vi "Test Clone Registration API.vi"() -> ()   [LabVIEW 2022 SP3, in "Serial-Com-Module.lvlib"]
doc: "Tester for the cloneable module registry VIs.\n_____\nBased on DQMH Project Template 6.1.0.94."
uses:
  Serial-Com-Module.lvlib
  Clone Registration.lvlib
panel:
  out "Empty?":bool
  out "First?":bool
  out "Module IDs":cluster{"Boolean":bool, "Numeric":i32}[](array[cluster])
  out "found?":bool
  out "replaced?":bool
  in  "Remove Module":bool
  in  "Add Module":bool
  in  "Module ID":i32
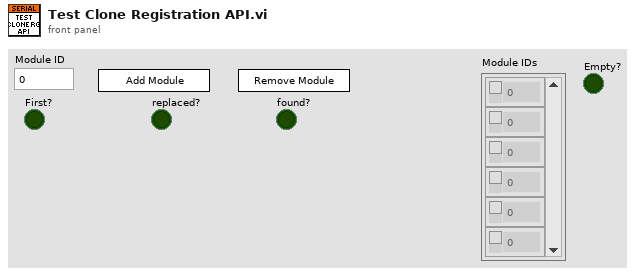
[diagram p1: front panel]
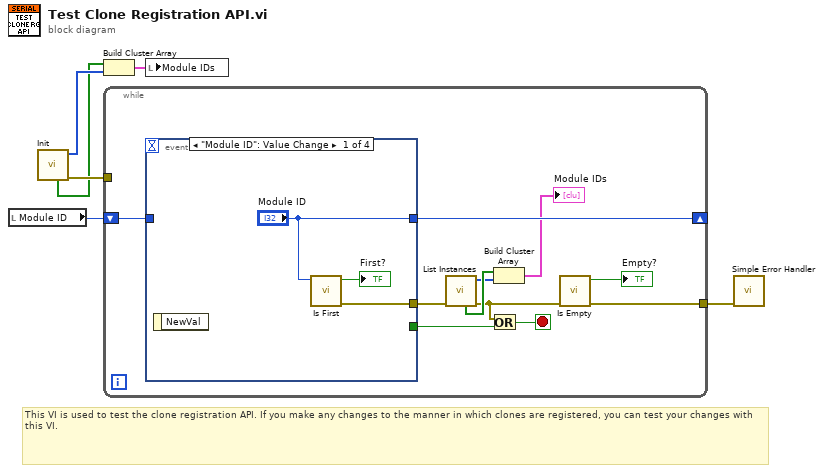
[diagram p0: block diagram]
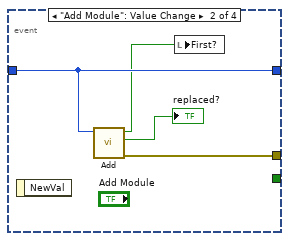
[diagram p2: hidden frame]
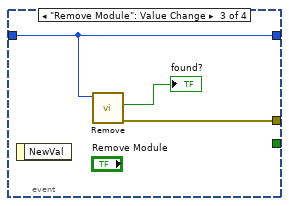
[diagram p3: hidden frame]
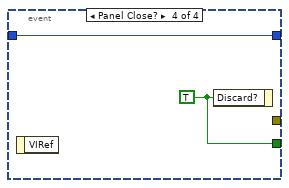
[diagram p4: hidden frame]
diagram:
  # "This VI is used to test the clone registration API. If you make any changes to the manner in which clones are registered, you can test your changes with this VI."
  n1 = local read "Module ID"() -> (w6:i32)
  n2 = call "Init.vi"() -> ("error out"=w2:errorcluster, "Module IDs"=w3:i32[], "First? (all)"=w1:bool[])  [unwired: 8 in, 1 out]
  n3 = Build Cluster Array(w1, w3) -> (w5:cluster{"First?":bool, "Module ID":i32}[])
  n4 = while {
    shift-right: [w16] -> _
    shift-left: w6 -> [w15]
    tunnel: w2 -> [_]
    tunnel: [w8] -> w4
    stop <- w14 stop-if-true
    n5 = event shown="[0] \"Module ID\": Value Change" {
      selector: _ -> [_ _ _ _]
      dyn-events: _ -> [_ _ _ _]
      timeout: _ -> [_ _ _ _]
      tunnel: [_ _ _ w29] -> w17
      tunnel: ["Module ID" w24 w25 w28] -> w16
      tunnel: w15 -> [_ w24 w25 w28]
      tunnel: [w18 w21 w27 _] -> w10
      event "Module ID": Value Change {
        n6 = event-data() -> ()  [unwired: 1 in, 1 out]
        n7 = call "Is First.vi"("Module ID"="Module ID") -> ("error out"=w18:errorcluster, "First?"=→"First?":bool)  [unwired: 9 in]
      }
      event "Add Module": Value Change {
        n8 = event-data() -> ()  [unwired: 1 in, 1 out]
        n9 = call "Add.vi"("Module ID"=w24) -> ("error out"=w21:errorcluster, "replaced?"=→"replaced?":bool, "First?"=w23:bool)  [unwired: 8 in]
        n10 = local write "First?"(w23) -> ()
      }
      event "Remove Module": Value Change {
        n11 = event-data() -> ()  [unwired: 1 in, 1 out]
        n12 = call "Remove.vi"("Module ID"=w25) -> ("error out"=w27:errorcluster, "empty"=→"found?":bool)  [unwired: 9 in]
      }
      event Panel Close? {
        w29 = TRUE ("Discard?")
        n13 = event-data() -> ()  [unwired: 1 in, 1 out]
        n14 = event-data("Discard?"=w29) -> ()  [unwired: 1 in, 1 out]
      }
    }
    n15 = call "List Instances.vi"("error in (no error)"=w10) -> ("error out"=w9:errorcluster, "Module IDs"=w11:i32[], "First?"=w12:bool[])  [unwired: 6 in, 2 out]
    n16 = Or(x=w9, y=w17) -> (x .or. y?=w14:bool)
    n17 = Build Cluster Array(w12, w11) -> (→"Module IDs":cluster{"First?":bool, "Module ID":i32}[])
    n18 = call "Is Empty.vi"("error in (no error)"=w9) -> ("error out"=w8:errorcluster, "Empty?"=→"Empty?":bool)  [unwired: 9 in]
  }
  n19 = local write "Module IDs"(w5) -> ()
  n20 = call <vilib>:"Simple Error Handler.vi"("error in (no error)"=w4) -> ()  [unwired: 4 in, 5 out]
